vi "MischerMonitor_Split_Cluster.vi"(0 "Mischer Monitor":T3) -> (1 "Mischer  Status":T2, 2 "Mischer  Control":T1)   [LabVIEW 2019]
uses:
  Mischer/Mischer-Cluster.ctl
  Mischer/Mischer-Status.ctl
  Mischer/Mischer-Control.ctl
panel:
  # "2"
  # "to Condenser"
  # "1"
  # "7"
  # "From Still"
  # "5"
  # "Mischer\nEinheit"
  # "12"
  # "Cold\nTrap"
  # "Dump"
  # "9"
  # "8"
  # "2"
  # "to Condenser"
  # "1"
  # "7"
  # "From Still"
  # "5"
  # "Mischer\nEinheit"
  # "12"
  # "Cold\nTrap"
  # "Dump"
  # "9"
  # "8"
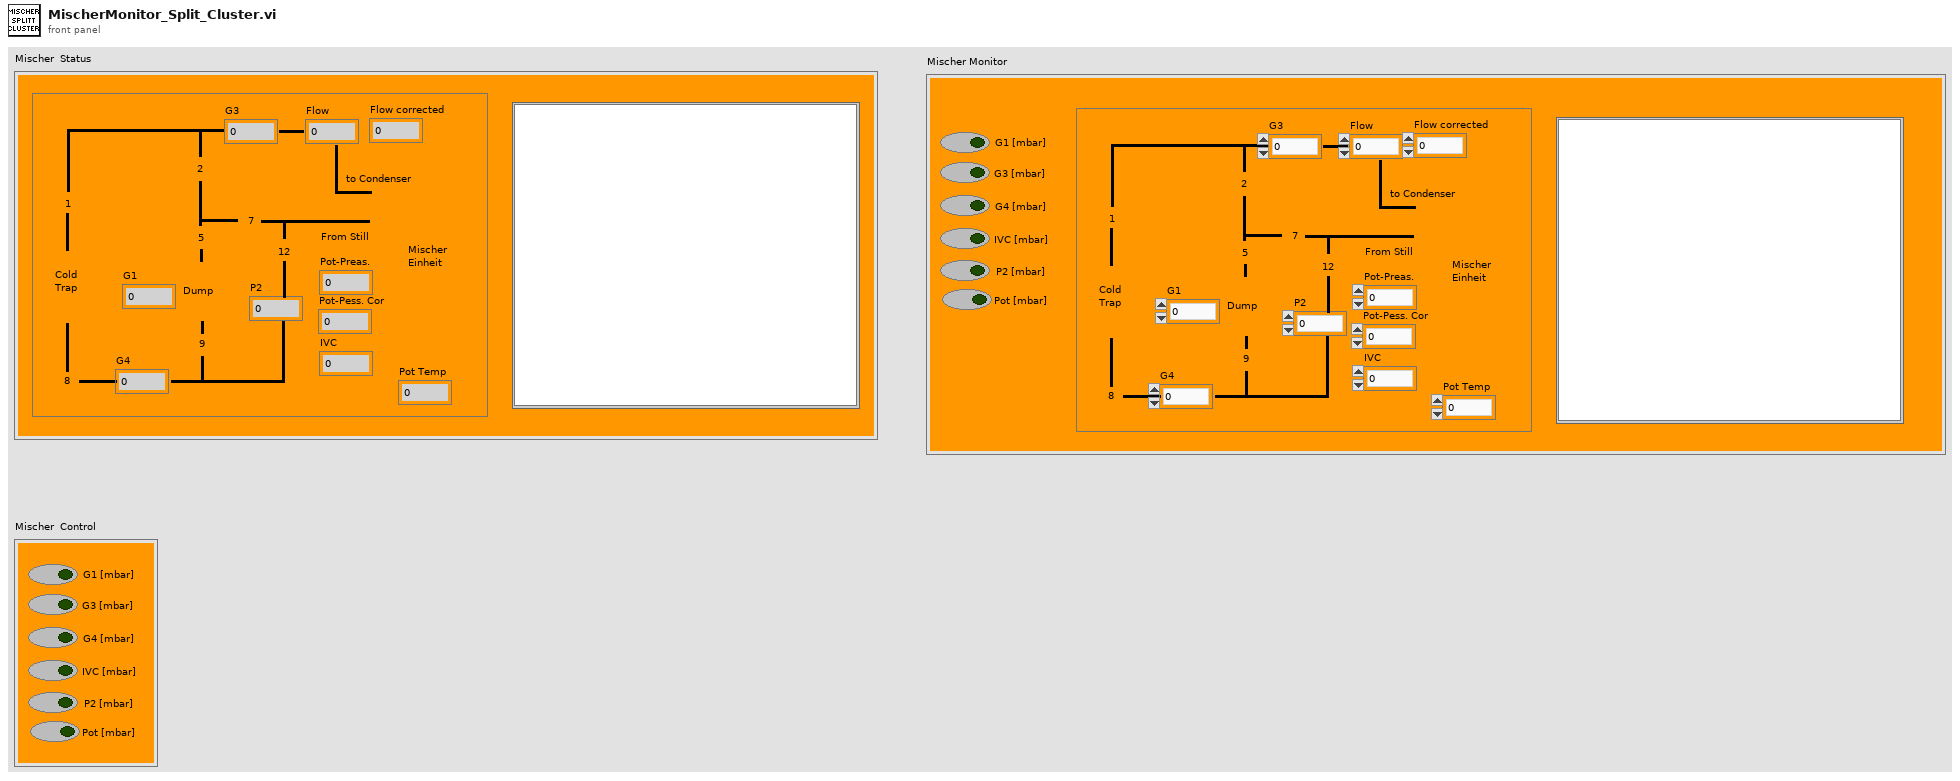
[diagram p1: front panel]
types:
  T1 = typedef "Mischer-Control.ctl" = cluster{"G1 [mbar]":bool, "G3 [mbar]":bool, "G4 [mbar]":bool, "IVC [mbar]":bool, "P2 [mbar] ":bool, "Pot [mbar]":bool}
  T2 = typedef "Mischer-Status.ctl" = cluster{"G4":dbl, "G1":dbl, "P2":dbl, "G3":dbl, "Flow":dbl, "Pot-Preas.":dbl, "IVC":dbl, "Flow corrected":dbl, "Pot-Pess. Cor":dbl, "Pot Temp":dbl, "Plot":dbl[][]}
  T3 = typedef "Mischer-Cluster.ctl" = cluster{"G4":dbl, "G1":dbl, "P2":dbl, "G3":dbl, "Flow":dbl, "Pot-Preas.":dbl, "IVC":dbl, "G1 [mbar]":bool, "G3 [mbar]":bool, "G4 [mbar]":bool, "IVC [mbar]":bool, "P2 [mbar] ":bool, "Flow corrected":dbl, "Pot-Pess. Cor":dbl, "Pot Temp":dbl, "Pot [mbar]":bool, "Plot":dbl[][]}
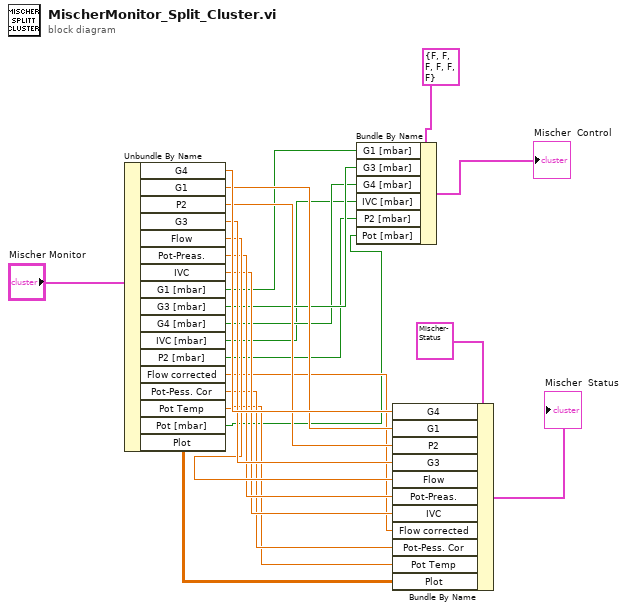
[diagram p0: block diagram]
diagram:
  n1 = Unbundle By Name("Mischer Monitor") -> ("G4"=w17:dbl, "G1"=w16:dbl, "P2"=w15:dbl, "G3"=w14:dbl, "Flow"=w13:dbl, "Pot-Preas."=w12:dbl, "IVC"=w11:dbl, "G1 [mbar]"=w6:bool, "G3 [mbar]"=w5:bool, "G4 [mbar]"=w4:bool, "IVC [mbar]"=w3:bool, "P2 [mbar]"=w2:bool, "Flow corrected"=w10:dbl, "Pot-Pess. Cor"=w9:dbl, "Pot Temp"=w8:dbl, "Pot [mbar]"=w1:bool, "Plot"=w7:dbl[][])
  n2 = Bundle By Name(cluster=T1 {"G1 [mbar]"=FALSE, "G3 [mbar]"=FALSE, "G4 [mbar]"=FALSE, "IVC [mbar]"=FALSE, "P2 [mbar] "=FALSE, "Pot [mbar]"=FALSE} ("Mischer  Control"), "G1 [mbar]"=w6, "G3 [mbar]"=w5, "G4 [mbar]"=w4, "IVC [mbar]"=w3, "P2 [mbar]"=w2, "Pot [mbar]"=w1) -> (→"Mischer  Control":T1)
  n3 = Bundle By Name(cluster=T2 {"G4"=0.0, "G1"=0.0, "P2"=0.0, "G3"=0.0, "Flow"=0.0, "Pot-Preas."=0.0, "IVC"=0.0, "Flow corrected"=0.0, "Pot-Pess. Cor"=0.0, "Pot Temp"=0.0, "Plot"=[]} ("Mischer  Status"), "G4"=w17, "G1"=w16, "P2"=w15, "G3"=w14, "Flow"=w13, "Pot-Preas."=w12, "IVC"=w11, "Flow corrected"=w10, "Pot-Pess. Cor"=w9, "Pot Temp"=w8, "Plot"=w7) -> (→"Mischer  Status":T2)
